vi "auto_ctrl_run_valve.vi"(4 "ref_reinit":refnum<vi>, 6 "ref_sp_turn":refnum<vi>, 7 "array_value_in":dbl[](array[numeric]) format="%.2f", 9 "level_set":dbl=80.0 format="%.1f", 10 "enable_auto_ctrl":bool caption="Auto Control", 11 "level":dbl=90.0 format="%.1f") -> (0 "turn_new":dbl format="%.3f", 1 "status":u32(colorbox), 5 "array_value_out":dbl[](array[numeric]))   [LabVIEW 2019]
doc: "This example demonstrates how to simulate a general PID controller."
uses:
  <vilib>/Analysis/baseanly.llb/Mean (DBL).vi
  <vilib>/addons/control/pid/pid.llb/PID (DBL).vi
  <vilib>/addons/control/pid/NI_PID_pid.lvlib
  <vilib>/Analysis/NI_AALBase.lvlib
panel:
  out "level_used":dbl format="%0.2f"
  in  "n_avg":u8=5
  in  "control_step":dbl=0.01 format="%#_13g"
  in  "turn_nominal":dbl=0.5 format="%.2f"
  in  "turn_max":dbl=2.0 format="%.2f"
  in  "turn_min":dbl=0.3 format="%.2f"
  out "MV":dbl format="%.1f"
  out "PID Range":cluster{"High":dbl, "Low":dbl} {"Low" format="%.1f"; "High" format="%.1f"}
  in  "PID gains":T1={"proportional gain (Kc)"=0.2, "integral time (Ti, min)"=0.5, "derivative time (Td, min)"=0.2} {"derivative time (Td, min)" format="%.4f"; "integral time (Ti, min)" format="%.4f"; "proportional gain (Kc)" format="%.3f"}
  # "gain = delta_turn / delta_level ~ 0.05 / 0.5 = 0.1"
  # "turn"
  # "turn"
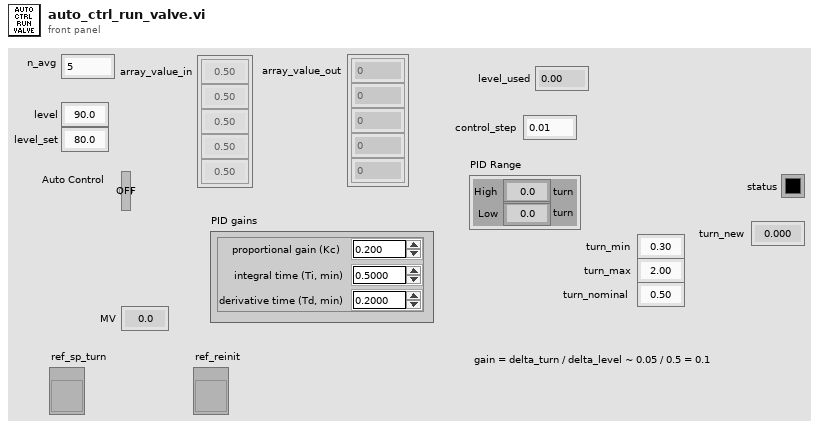
[diagram p1: front panel]
types:
  T1 = cluster{"proportional gain (Kc)":dbl, "integral time (Ti, min)":dbl, "derivative time (Td, min)":dbl}
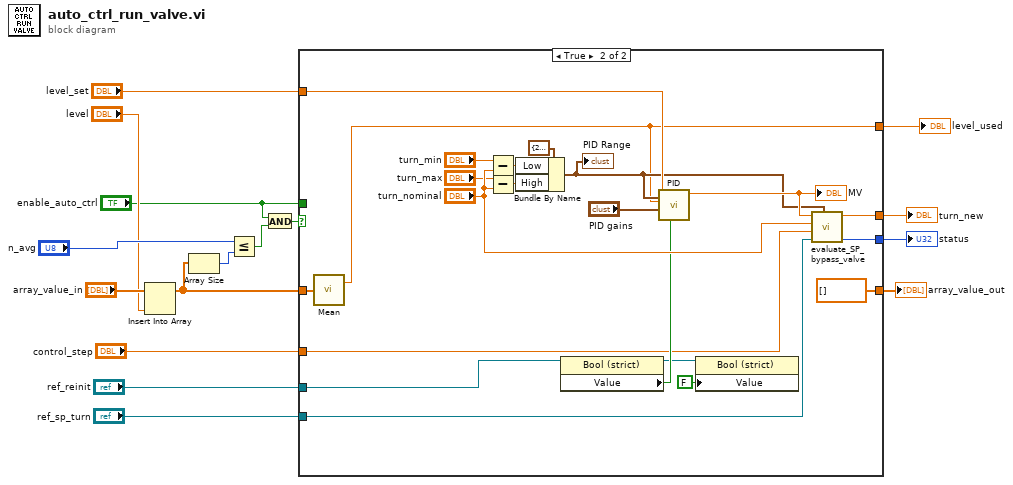
[diagram p0: block diagram]
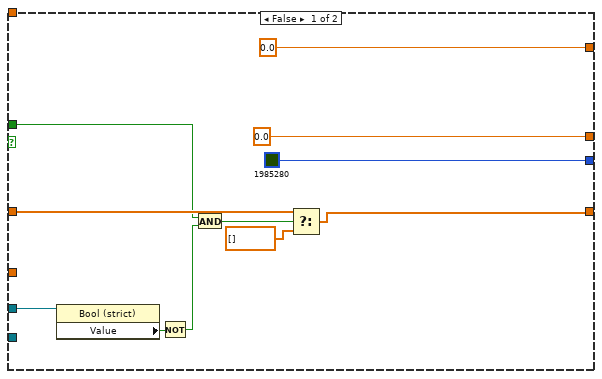
[diagram p2: hidden frame]
diagram:
  n1 = Insert Into Array(array="array_value_in", new element="level") -> (w3:dbl[])  [unwired: 1 in]
  n2 = Array Size(array=w3) -> (size(s)=w9:i32)
  n3 = Less Or Equal?(x="n_avg", y=w9) -> (x <= y?=w7:bool)
  n4 = And(x="enable_auto_ctrl", y=w7) -> (x .and. y?=w11:bool)
  n5 = case shown="True" w11 {
    tunnel: [0.0 ("F_O_new") w46] -> w16
    tunnel: [u32 1985280 ("alarm_status") w48] -> w15
    tunnel: "level_set" -> [_ w44]
    tunnel: "ref_sp_turn" -> [_ w47]
    tunnel: "ref_reinit" -> [w21 w42]
    tunnel: "control_step" -> [_ w31]
    tunnel: [w23 dbl[] [] ("array_value_in")] -> w6
    tunnel: w3 -> [w24 w30]
    tunnel: [0.0 ("mean") w28] -> w2
    tunnel: "enable_auto_ctrl" -> [w17 _]
    frame False {
      n6 = property class="Bool (strict)"(reference=w21) -> ("Value"=w20:bool)  [unwired: 1 in, 2 out]
      n7 = Not(x=w20) -> (.not. x?=w18:bool)
      n8 = And(x=w17, y=w18) -> (x .and. y?=w19:bool)
      n9 = Select(t=w24, s=w19, f=dbl[] []) -> (s? t:f=w23:dbl[])
    }
    frame True {
      n10 = call-poly <vilib>:"Mean.vi"("X"=w30) -> ("mean"=w28:dbl)  [unwired: 1 out]
      n11 = Subtract(x="turn_min", y="turn_nominal") -> (x-y=w36:dbl)
      n12 = Subtract(x="turn_max", y="turn_nominal") -> (x-y=w37:dbl)
      n13 = Bundle By Name(cluster=cluster{"High":dbl, "Low":dbl} {"High"=20.0, "Low"=-20.0} ("PID Range"), "Low"=w36, "High"=w37) -> (w32:cluster{"High":dbl, "Low":dbl})
      "PID Range" <- w32
      n14 = property class="Bool (strict)"(reference=w42) -> (reference out=w40:refnum<vi>, "Value"=w41:bool)  [unwired: 1 in, 1 out]
      n15 = call-poly <vilib>:"PID.vi"("reinitialize? (F)"=w41, "output range"=w32, "PID gains"="PID gains", "process variable"=w28, "setpoint"=w44) -> ("output"=w43:dbl)  [unwired: 5 in, 1 out]
      "MV" <- w43
      n16 = property class="Bool (strict)"(reference=w40, "Value"=FALSE) -> ()  [unwired: 1 in, 2 out]
      n17 = call "evaluate_SP_bypass_valve.vi"("PID Range"=w32, "ref_sp_ch1"=w47, "control_step"=w31, "F_org"="turn_nominal", "control"=w43) -> ("status"=w48:u32, "F_new"=w46:dbl)  [unwired: 5 in]
    }
  }
  "turn_new" <- w16
  "status" <- w15
  "array_value_out" <- w6
  "level_used" <- w2
